vi "Z.关闭Log.vi"(8 "error in (no error)":errorcluster, 11 "Module ID":i32=-1) -> (0 "error out":errorcluster)   [LabVIEW 2020, in "Log.lvlib"]
uses:
  Log.lvlib
  Log.lvlibp
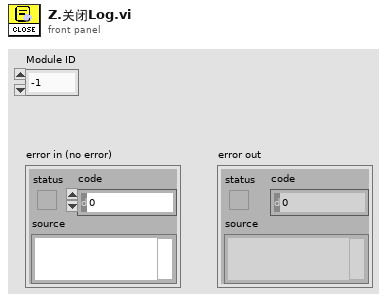
[diagram p1: front panel]
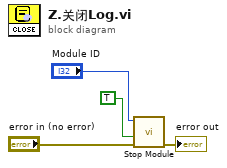
[diagram p0: block diagram]
diagram:
  n1 = call "Stop Module.vi"("error in (no error)"="error in (no error)", "Wait for Module to stop? (F)"=TRUE, "Module ID"="Module ID") -> ("error out"=→"error out":errorcluster)  [unwired: 8 in]
